vi "Force Odd or Even.vi"(1 "Parity (odd)":enum16{"Odd", "Even"}(ring), 2 "input":i32) -> (0 "output":i32)   [LabVIEW 2022 SP3]
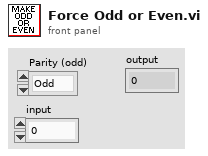
[diagram p1: front panel]
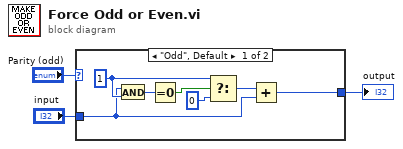
[diagram p0: block diagram]
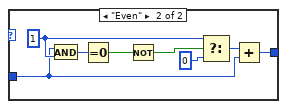
[diagram p2: hidden frame]
diagram:
  n1 = case shown="\"Odd\", Default" "Parity (odd)" {
    tunnel: "input" -> [w5 w12]
    tunnel: [w4 w11] -> w1
    frame "Odd", Default {
      w7 = 1 ("y")
      n2 = And(x=w5, y=w7) -> (x .and. y?=w6:i32)
      n3 = Equal To 0?(x=w6) -> (x = 0?=w10:bool)
      n4 = Select(t=w7, s=w10, f=0) -> (s? t:f=w9:i32)
      n5 = Add(x=w9, y=w5) -> (x+y=w4:i32)
    }
    frame "Even" {
      w14 = 1 ("y")
      n6 = And(x=w12, y=w14) -> (x .and. y?=w13:i32)
      n7 = Equal To 0?(x=w13) -> (x = 0?=w17:bool)
      n8 = Not(x=w17) -> (.not. x?=w18:bool)
      n9 = Select(t=w14, s=w18, f=0) -> (s? t:f=w16:i32)
      n10 = Add(x=w16, y=w12) -> (x+y=w11:i32)
    }
  }
  "output" <- w1
